vi "ErrorHandler.vi"(8 "error in (no error)":errorcluster, 10 "[error source]":string, 11 "[error code]":i32) -> (0 "error out":errorcluster, 3 "error?":bool)   [LabVIEW 2013]
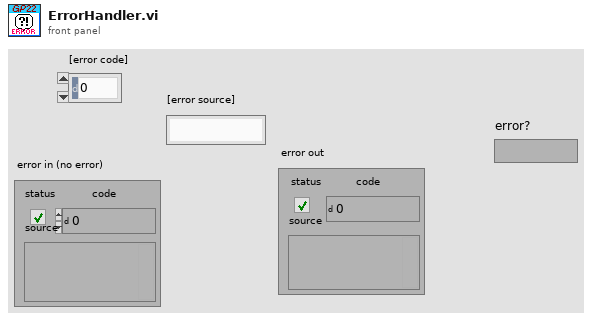
[diagram p1: front panel]
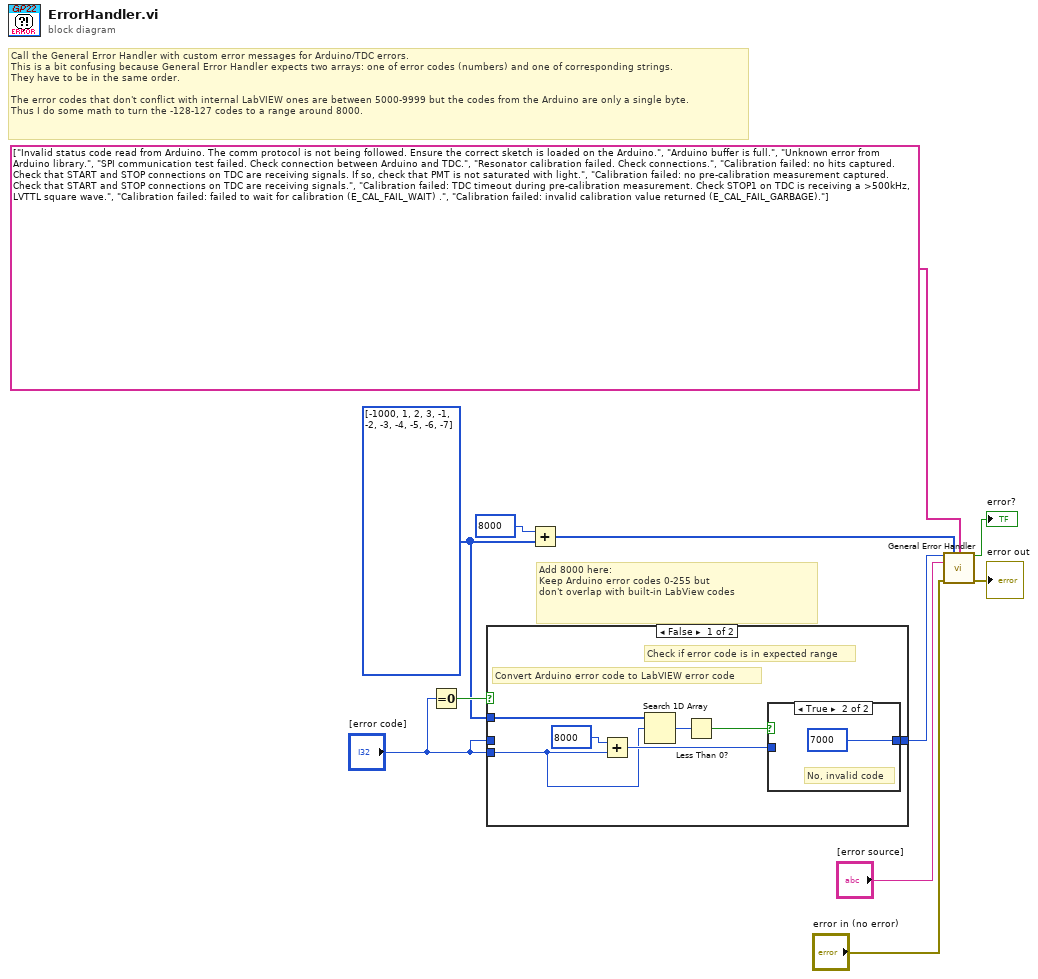
[diagram p0: block diagram]
diagram:
  w3 = i32[] [-1000, 1, 2, 3, -1, -2, -3, -4, -5, -6, -7]
  # "Call the General Error Handler with custom error messages for Arduino/TDC errors.\nThis is a bit confusing because General Error Handler expects two arrays: one of error codes (numbers) and one of corresponding strings.\nThey have to be in the same order.\n\nThe error codes that don't conflict with internal LabVIEW ones are between 5000-9999 but the codes from the Arduino are only a single byte.\nThus I do some math to turn the -128-127 codes to a range around 8000."
  # "Add 8000 here:\nKeep Arduino error codes 0-255 but\ndon't overlap with built-in LabView codes"
  n1 = Equal To 0?(x="[error code]") -> (x = 0?=w4:bool)
  n2 = case shown="False" w4 {
    tunnel: [w14 w21] -> w1
    tunnel: "[error code]" -> [_ w21]
    tunnel: w3 -> [w16 _]
    tunnel: "[error code]" -> [w12 _]
    frame False {
      # "Convert Arduino error code to LabVIEW error code"
      # "Check if error code is in expected range"
      n3 = Add(x=8000, y=w12) -> (x+y=w13:i32)
      n4 = Search 1D Array(1D array=w16, element=w12) -> (index of element=w18:i32)  [unwired: 1 in]
      n5 = Less Than 0?(x=w18) -> (x < 0?=w15:bool)
      n6 = case shown="True" w15 {
        tunnel: [w19 7000] -> w14
        tunnel: w13 -> [w19 _]
        frame False {
          # "Yes, valid code"
        }
        frame True {
          # "No, invalid code"
        }
      }
    }
    frame True {
      # "Error code is 0, E_OK. Don't do any math."
    }
  }
  n7 = Add(x=8000, y=w3) -> (x+y=w6:i32[])
  n8 = call <vilib>:"General Error Handler.vi"("[error code] (0)"=w1, "[user-defined codes]"=w6, "[user-defined descriptions]"=string[] ["Invalid status code read from Arduino. The comm protocol is not being followed. Ensure the correct sketch is loaded on the Arduino.", "Arduino buffer is full.", "Unknown error from Arduino library.", "SPI communication test failed. Check connection between Arduino and TDC.", "Resonator calibration failed. Check connections.", "Calibration failed: no hits captured. Check that START and STOP connections on TDC are receiving signals. If so, check that PMT is not saturated with light.", "Calibration failed: no pre-calibration measurement captured. Check that START and STOP connections on TDC are receiving signals.", "Calibration failed: TDC timeout during pre-calibration measurement. Check STOP1 on TDC is receiving a >500kHz, LVTTL square wave.", "Calibration failed: failed to wait for calibration (E_CAL_FAIL_WAIT) .", "Calibration failed: invalid calibration value returned (E_CAL_FAIL_GARBAGE)."], "[error source] (\" \")"="[error source]", "error in (no error)"="error in (no error)") -> ("error?"=→"error?":bool, "error out"=→"error out":errorcluster)  [unwired: 6 in, 3 out]
